vi "check_py_session.vi"(4 "error in":errorcluster, 6 "Request data":variant, 7 "Python session in":refnum<k35>) -> (0 "error out":errorcluster, 2 "Response data":variant, 3 "Python session out":refnum<k35>)   [LabVIEW 2018]
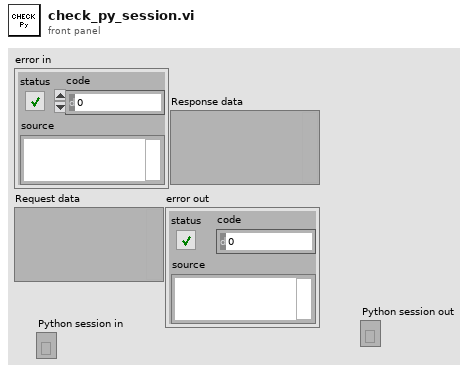
[diagram p1: front panel]
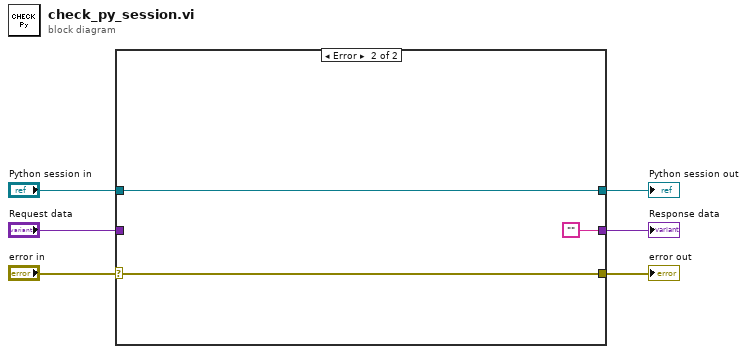
[diagram p0: block diagram]
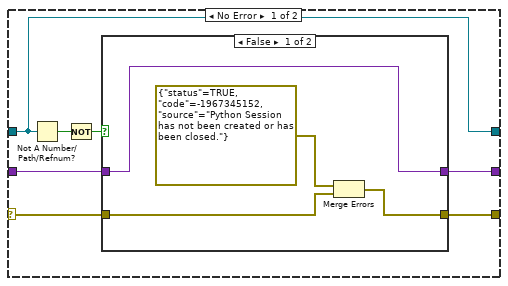
[diagram p2: hidden frame]
diagram:
  n1 = case shown="Error" "error in" {
    selector: "error in" -> [w10 w22]
    tunnel: [w13 w22] -> w5
    tunnel: "Request data" -> [w9 _]
    tunnel: [w8 ""] -> w3
    tunnel: "Python session in" -> [w7 w20]
    tunnel: [w7 w20] -> w1
    frame No Error {
      n2 = Not A Number/Path/Refnum?(number/path/refnum=w7) -> (NaN/Path/Refnum?=w12:bool)
      n3 = Not(x=w12) -> (.not. x?=w11:bool)
      n4 = case shown="False" w11 {
        tunnel: w10 -> [w17 w18]
        tunnel: [w15 w18] -> w13
        tunnel: w9 -> [w14 w19]
        tunnel: [w14 w19] -> w8
        frame False {
          n5 = Merge Errors(errorcluster {"status"=TRUE, "code"=-1967345152, "source"="Python Session has not been created or has been closed."} ("error constant"), w17) -> (w15:errorcluster)
        }
        frame True {
        }
      }
    }
    frame Error {
    }
  }
  "Response data" <- w3
  "error out" <- w5
  "Python session out" <- w1
